vi "RndGenerator.vi"() -> (0 "Double digit":u64, 3 "Decimal integer string":string)   [LabVIEW 2023]
uses:
  <vilib>/numeric/Random Number (Range) U64.vi
  <vilib>/numeric/sub_Random U32.vi
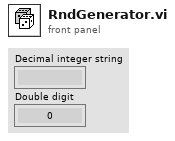
[diagram p1: front panel]
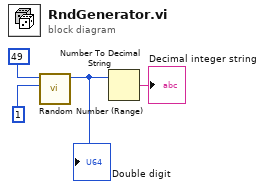
[diagram p0: block diagram]
diagram:
  n1 = call-poly <vilib>:"Random Number (Range).vi"("lower bound (0)"=u64 1, "upper bound (100)"=u64 49) -> ("number"=w2:u64)  [unwired: 9 in]
  "Double digit" <- w2
  n2 = Number To Decimal String(number=w2) -> (decimal integer string=→"Decimal integer string":string)  [unwired: 1 in]
